vi "Find Incremental File.vi"(4 "error in (no error)":errorcluster, 6 "Filename (empty)":string, 7 "Folder Path":path) -> (0 "error out":errorcluster, 2 "No Match?":bool, 3 "Unique Incremental Path":path)   [LabVIEW 2011]
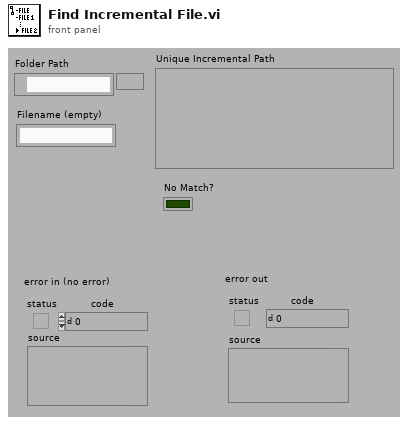
[diagram p1: front panel]
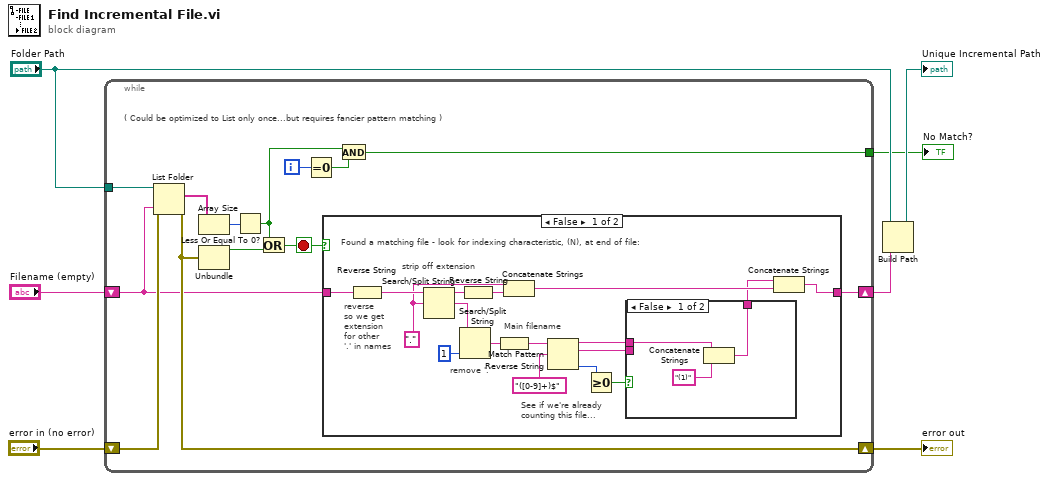
[diagram p0: block diagram]
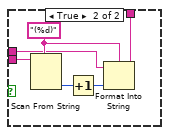
[diagram p2: hidden frame]
diagram:
  n1 = while {
    tunnel: "Folder Path" -> [w20]
    shift-right: [w12] -> w4
    shift-left: "Filename (empty)" -> [w13]
    shift-right: [w16] -> w6
    shift-left: "error in (no error)" -> [w19]
    tunnel: [w8] -> w1
    i -> [w10]
    stop <- w14 stop-if-true
    # "( Could be optimized to List only once...but requires fancier pattern matching )"
    n2 = List Folder(path=w20, pattern=w13, error in=w19) -> (filenames=w18:string[], error out=w16:errorcluster)  [unwired: 3 out]
    n3 = Array Size(array=w18) -> (size(s)=w17:i32)
    n4 = Unbundle(w16) -> ("status"=w15:bool)  [unwired: 2 out]
    n5 = Less Or Equal To 0?(x=w17) -> (x <= 0?=w11:bool)
    n6 = Or(x=w11, y=w15) -> (x .or. y?=w14:bool)
    n7 = Equal To 0?(x=w10) -> (x = 0?=w9:bool)
    n8 = case shown="False" w14 {
      tunnel: w13 -> [w37 w47]
      tunnel: [w29 w47] -> w12
      frame False {
        w31 = "."
        # "Main filename"
        # "See if we're already\ncounting this file..."
        # "Found a matching file - look for indexing characteristic, (N), at end of file:"
        # "remove '.'"
        # "reverse\nso we get\nextension\nfor other\n'.' in names"
        # "strip off extension"
        n9 = Reverse String(1:w37) -> (0:w36:string)
        n10 = Search/Split String(string=w36, search string/char (-)=w31) -> (substring before match=w33:string, match + rest of string=w35:string)  [unwired: 2 out]
        n11 = Search/Split String(string=w35, offset (0)=1) -> (match + rest of string=w28:string)  [unwired: 3 out]
        n12 = Reverse String(1:w33) -> (0:w32:string)
        n13 = Reverse String(1:w28) -> (0:w27:string)
        n14 = Concatenate Strings(w31, w32) -> (w30:string)
        n15 = Match Pattern(string=w27, regular expression="([0-9]+)$") -> (before substring=w23:string, match substring=w24:string, offset past match=w25:i32)  [unwired: 2 out]
        n16 = Greater Or Equal To 0?(x=w25) -> (x >= 0?=w21:bool)
        n17 = case shown="False" w21 {
          tunnel: w24 -> [_ w46]
          tunnel: w23 -> [w40 w42]
          tunnel: [w38 w41] -> w22
          frame False {
            n18 = Concatenate Strings(w40, "(1)") -> (w38:string)
          }
          frame True {
            w43 = "(%d)"
            n19 = Scan From String(format string=w43, input string=w46) -> (output 1=w45:i32)  [unwired: 2 in, 4 out]
            n20 = Increment(x=w45) -> (x+1=w44:i32)
            n21 = Format Into String(format string=w43, initial string=w42, w44) -> (resulting string=w41:string)  [unwired: 1 in, 1 out]
          }
        }
        n22 = Concatenate Strings(w22, w30) -> (w29:string)
      }
      frame True {
        # "File match NOT found (or error) - stop the loop and use this Filename..."
      }
    }
    n23 = And(x=w11, y=w9) -> (x .and. y?=w8:bool)
  }
  "error out" <- w6
  "No Match?" <- w1
  n24 = Build Path(base path="Folder Path", name or relative path=w4) -> (appended path=→"Unique Incremental Path":path)
